vi "test shift.vi"() -> ()   [LabVIEW 2019]
panel:
  in  "Numeric":i32=1000000
  out "iter per ms":dbl
  out "dt":u32
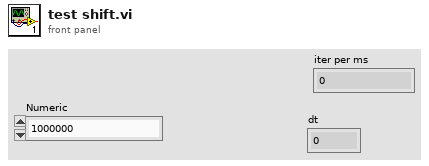
[diagram p1: front panel]
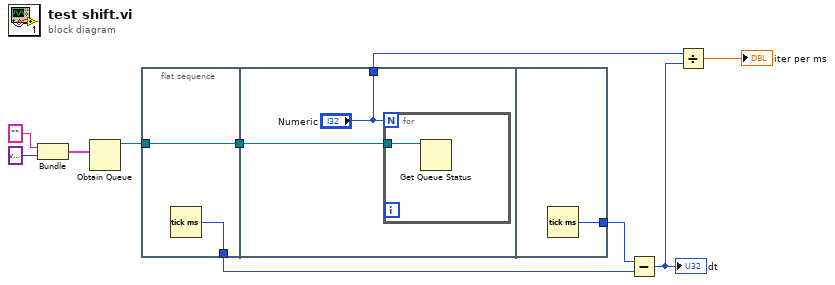
[diagram p0: block diagram]
diagram:
  n1 = Bundle("", variant) -> (w10:cluster{string, variant})  [unwired: 1 in]
  n2 = Obtain Queue(element data type=w10) -> (queue out=w6:refnum<queue>)  [unwired: 4 in, 2 out]
  n3 = flat-sequence {
    tunnel: [w12] -> w7
    tunnel: w6 -> [w12]
    tunnel: [w11] -> w4
    tunnel: w7 -> [w14]
    tunnel: ["Numeric"] -> w2
    tunnel: [w16] -> w5
    frame #0 {
      n4 = Tick Count (ms)() -> (millisecond timer value=w11:u32)
    }
    frame #1 {
      n5 = for {
        N: "Numeric" -> [_]
        tunnel: w14 -> [w15]
        n6 = Get Queue Status(queue=w15) -> ()  [unwired: 2 in, 8 out]
      }
    }
    frame #2 {
      n7 = Tick Count (ms)() -> (millisecond timer value=w16:u32)
    }
  }
  n8 = Subtract(x=w5, y=w4) -> (x-y=w3:u32)
  "dt" <- w3
  n9 = Divide(x=w2, y=w3) -> (x/y=→"iter per ms":dbl)
